vi "Comments.Add Wiring Description.vi"(8 "error in (no error)":errorcluster, 11 "Control Experiment in":refnum<class "Control Experiment.lvclass">) -> (0 "error out":errorcluster, 2 "Wiring Description":string, 3 "Control Experiment out":refnum<class "Control Experiment.lvclass">)   [LabVIEW 2019, in "Control Experiment.lvclass"]
uses:
  Control Experiment.lvclass
  <userlib>/LevyLab/Krohn Hite 7008/Inst.Krohn-Hite-7008/Inst.Krohn-Hite-7008.lvclass
  Control Experiment.lvclass/Control Experiment.ctl
  <userlib>/LevyLab/PLYM/YAML.lvclass
  C:/Program Files (x86)/National Instruments/LabVIEW 2019/user.lib/LevyLab/Instrument Framework/Instrument Types/Amplifier/Instrument.Amplifier.lvclass
  C:/Program Files (x86)/National Instruments/LabVIEW 2019/user.lib/LevyLab/Instrument Framework/Instrument/Instrument.lvclass
  C:/Program Files (x86)/National Instruments/LabVIEW 2019/vi.lib/JKI/JKI SMO/SMO/SMO.lvclass
panel:
  out "Numeric":i32
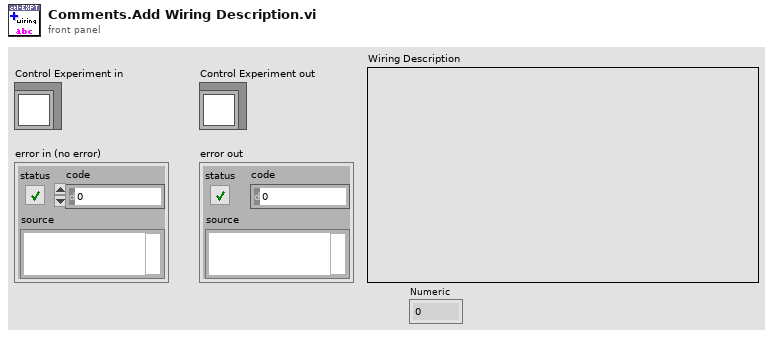
[diagram p1: front panel]
types:
  T1 = typedef "KH7008.lvlib/allChannelProperties--Array.ctl" = T2[]
  T2 = typedef "KH7008.lvlib/channelProperties--Cluster.ctl" = cluster{"channel":T3, "gain":T4, "input":T5, "shunt":T6, "couple":T7, "filter":T8}
  T3 = typedef "KH7008.lvlib/channel--numeric.ctl" = u16
  T4 = typedef "KH7008.lvlib/gain--enum.ctl" = enum16{"1", "10", "100", "1000"}
  T5 = typedef "KH7008.lvlib/input--enum.ctl" = enum16{"OFF", "SE+", "SE-", "DIFF"}
  T6 = typedef "KH7008.lvlib/shunt--enum.ctl" = enum16{"Open", "50", "500", "5k", "50k", "10M"}
  T7 = typedef "KH7008.lvlib/couple--enum.ctl" = enum16{"AC", "DC"}
  T8 = typedef "KH7008.lvlib/filter--enum.ctl" = enum16{"OFF", "ON"}
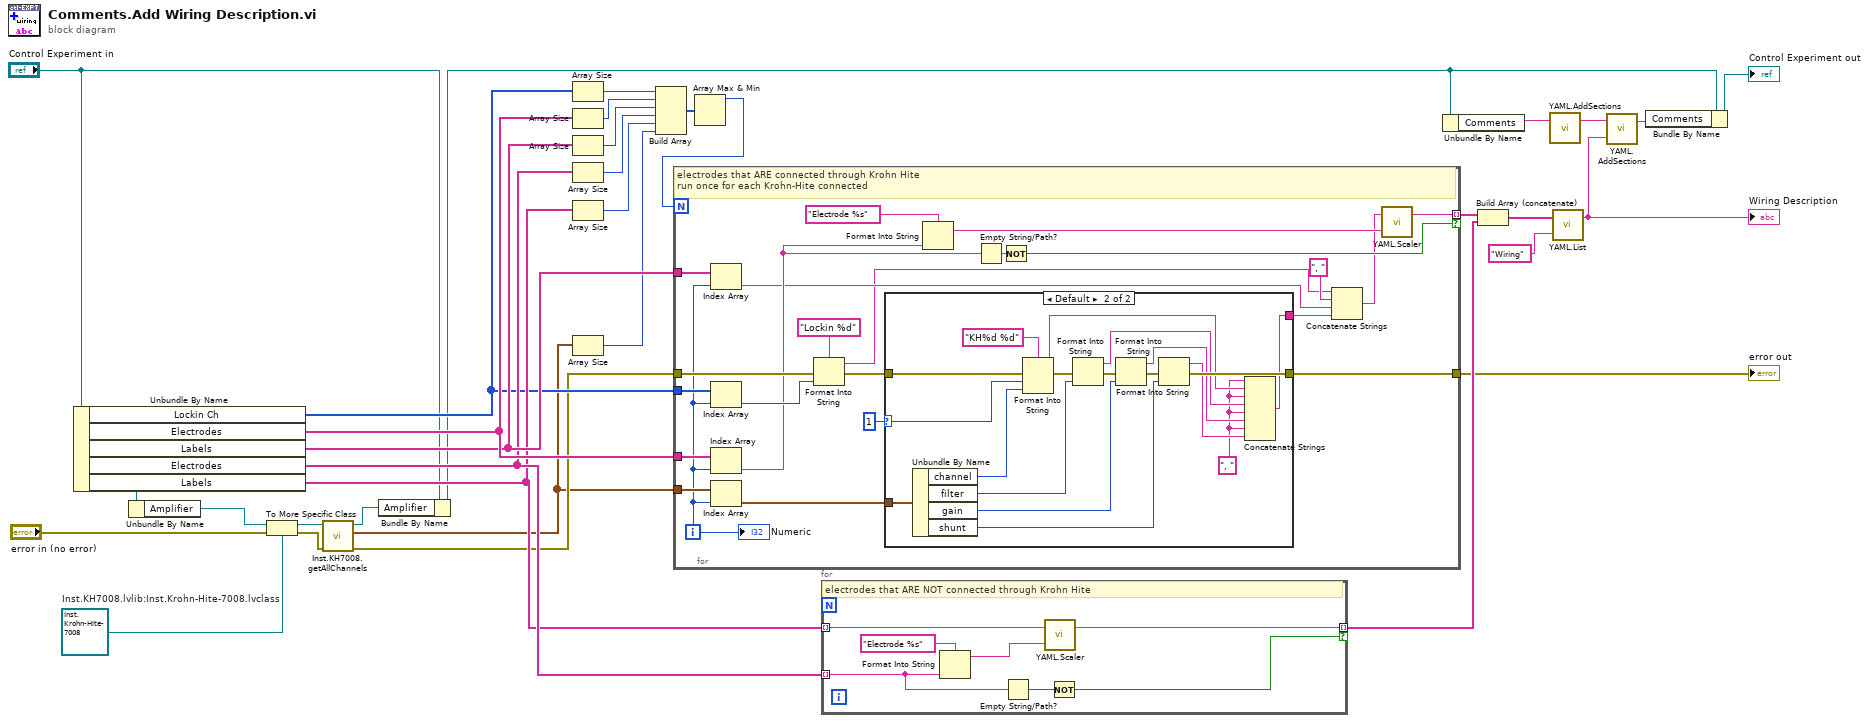
[diagram p0: block diagram]
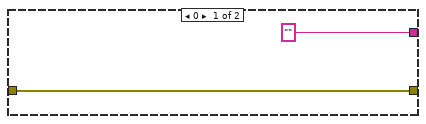
[diagram p2: hidden frame]
diagram:
  w10 = refnum<class "Inst.Krohn-Hite-7008.lvclass"> refnum  # Inst.KH7008.lvlib:Inst.Krohn-Hite-7008.lvclass
  n1 = Unbundle By Name("Control Experiment in") -> ("Lockin Ch"=w16:i32[], "Electrodes"=w23:string[], "Labels"=w22:string[], "Electrodes"=w21:string[], "Labels"=w20:string[])
  n2 = Unbundle By Name("Control Experiment in") -> ("Amplifier"=w1:refnum<class "Instrument.Amplifier.lvclass">)
  n3 = To More Specific Class(target class=w10, reference=w1, error in="error in (no error)") -> (specific class reference=w9:refnum<class "Inst.Krohn-Hite-7008.lvclass">, error out=w8:errorcluster)
  n4 = call-dynamic "Inst.KH7008.getAllChannels.vi"("error in (no error)"=w8, "Inst.Krohn-Hite-7008 in"=w9) -> ("error out"=w6:errorcluster, "allChannelProperties"=w5:T1, "Inst.Krohn-Hite-7008 out"=w4:refnum<class "Inst.Krohn-Hite-7008.lvclass">)  [unwired: 7 in]
  n5 = Bundle By Name(cluster="Control Experiment in", "Amplifier"=w4) -> (w2:refnum<class "Control Experiment.lvclass">)
  n6 = Array Size(array=w16) -> (size(s)=w19:i32)
  n7 = Array Size(array=w23) -> (size(s)=w18:i32)
  n8 = Array Size(array=w22) -> (size(s)=w17:i32)
  n9 = Array Size(array=w21) -> (size(s)=w15:i32)
  n10 = Array Size(array=w20) -> (size(s)=w14:i32)
  n11 = Array Size(array=w5) -> (size(s)=w13:i32)
  n12 = Build Array(w19, w18, w17, w15, w14, w13) -> (w12:i32[])
  n13 = Array Max & Min(array=w12) -> (max value=w11:i32)  [unwired: 3 out]
  n14 = for {
    N: w11 -> [_]
    tunnel: w16 -> [w45]
    tunnel: w23 -> [w51]
    tunnel: w22 -> [w44]
    tunnel: [w48] -> w27 mode=indexing if=w54
    tunnel: w6 -> [w50]
    tunnel: [w46] -> w25
    tunnel: w5 -> [w53]
    i -> [w35]
    # "electrodes that ARE connected through Krohn Hite\nrun once for each Krohn-Hite connected"
    n15 = Index Array(array=w44, index=w35) -> (element=w37:string)
    n16 = Index Array(array=w45, index=w35) -> (element=w43:i32)
    n17 = Index Array(array=w51, index=w35) -> (element=w42:string)
    n18 = Index Array(array=w53, index=w35) -> (element=w41:T2)
    n19 = Format Into String(format string="Lockin %d", error in=w50, w43) -> (resulting string=w36:string, error out=w56:errorcluster)  [unwired: 1 in]
    n20 = case shown="Default" 1 {
      selector: 1 -> [_ w59]
      tunnel: w56 -> [w58 w73]
      tunnel: ["" w60] -> w38
      tunnel: [w58 w67] -> w46
      tunnel: w41 -> [_ w66]
      frame 0 {
      }
      frame Default {
        w61 = ", "
        n21 = Unbundle By Name(w66) -> ("channel"=w68:T3, "filter"=w72:T8, "gain"=w71:T4, "shunt"=w70:T6)
        n22 = Format Into String(format string="KH%d %d", error in=w73, w59, w68) -> (resulting string=w62:string, error out=w76:errorcluster)  [unwired: 1 in]
        n23 = Format Into String(error in=w76, w72) -> (resulting string=w63:string, error out=w75:errorcluster)  [unwired: 2 in]
        n24 = Format Into String(error in=w75, w71) -> (resulting string=w64:string, error out=w74:errorcluster)  [unwired: 2 in]
        n25 = Format Into String(error in=w74, w70) -> (resulting string=w65:string, error out=w67:errorcluster)  [unwired: 2 in]
        n26 = Concatenate Strings(w61, w62, w61, w63, w61, w64, w61, w65) -> (w60:string)
      }
    }
    n27 = Format Into String(format string="Electrode %s", w42) -> (resulting string=w49:string)  [unwired: 2 in, 1 out]
    n28 = Empty String/Path?(string/path=w42) -> (empty?=w55:bool)
    n29 = Not(x=w55) -> (.not. x?=w54:bool)
    n30 = Concatenate Strings(w36, ", ", w37, w38) -> (w40:string)
    n31 = call <userlib>:"YAML.Scaler.vi"("Key"=w49, "Scaler"=w40) -> ("Output"=w48:string)  [unwired: 1 in]
    "Numeric" <- w35
  }
  "error out" <- w25
  n32 = for {
    tunnel: [w77] -> w28 mode=indexing if=w81
    tunnel: w20 -> [w78] mode=indexing
    tunnel: w21 -> [w83] mode=indexing
    # "electrodes that ARE NOT connected through Krohn Hite"
    n33 = Format Into String(format string="Electrode %s", w83) -> (resulting string=w79:string)  [unwired: 2 in, 1 out]
    n34 = Empty String/Path?(string/path=w83) -> (empty?=w82:bool)
    n35 = call <userlib>:"YAML.Scaler.vi"("Key"=w79, "Scaler"=w78) -> ("Output"=w77:string)  [unwired: 1 in]
    n36 = Not(x=w82) -> (.not. x?=w81:bool)
  }
  n37 = Unbundle By Name(w2) -> ("Comments"=w30:string)
  n38 = Build Array (concatenate)(w27, w28) -> (w29:string[])
  n39 = call <userlib>:"YAML.AddSections.vi"("Section 1"=w30) -> ("Output"=w32:string)  [unwired: 2 in]
  n40 = call <userlib>:"YAML.List.vi"("Key"="Wiring" ("string"), "lines"=w29) -> ("Output"=w24:string)  [unwired: 1 in]
  "Wiring Description" <- w24
  n41 = call <userlib>:"YAML.AddSections.vi"("Section 2"=w24, "Section 1"=w32) -> ("Output"=w33:string)  [unwired: 1 in]
  n42 = Bundle By Name(cluster=w2, "Comments"=w33) -> (→"Control Experiment out":refnum<class "Control Experiment.lvclass">)
